vi "FTW-ProjectItem-OwningProject.vi"(0 "ProjectItem":refnum<vi>, 11 "error in":errorcluster) -> (4 "ProjectItem out":refnum<vi>, 6 "Project":refnum<vi>, 15 "error out":errorcluster)   [LabVIEW 2012]
panel:
  # "Inputs"
  # "Outputs"
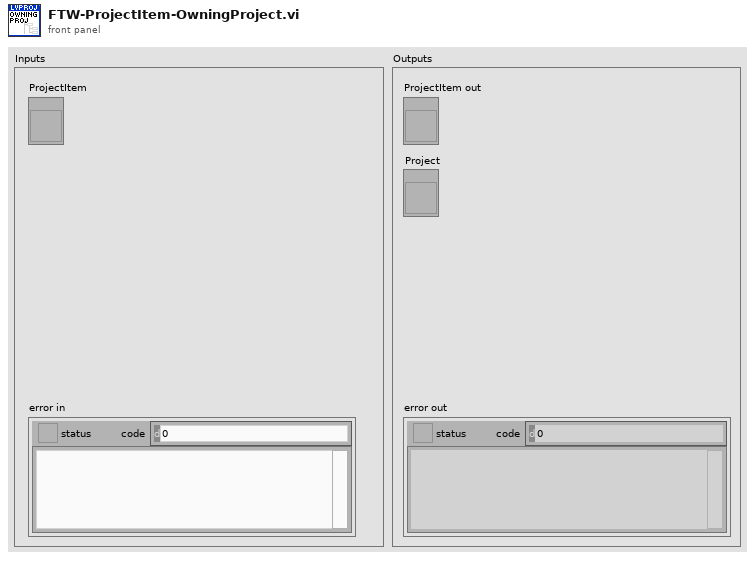
[diagram p1: front panel]
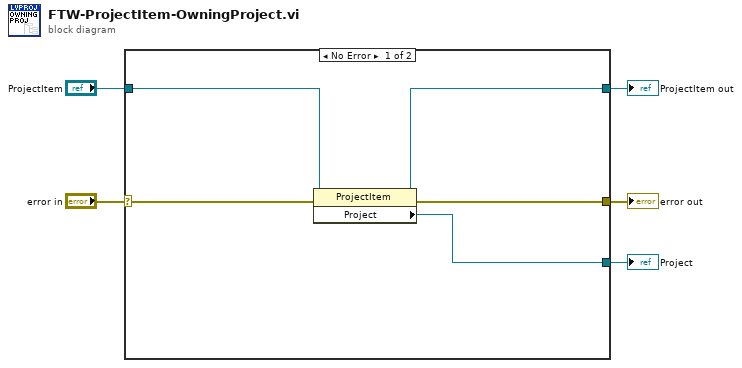
[diagram p0: block diagram]
diagram:
  n1 = case shown="No Error" "error in" {
    selector: "error in" -> [w10 w12]
    tunnel: [w7 w12] -> w5
    tunnel: "ProjectItem" -> [w8 w11]
    tunnel: [w9 w11] -> w2
    tunnel: [w6 _] -> w1
    frame No Error {
      n2 = property class="ProjectItem"(reference=w8, error in=w10) -> (reference out=w9:refnum<vi>, error out=w7:errorcluster, "Project"=w6:refnum<vi>)
    }
    frame Error {
    }
  }
  "error out" <- w5
  "ProjectItem out" <- w2
  "Project" <- w1
